vi "Main.vi"() -> ()   [LabVIEW 2019]
uses:
  Typedefs/#enum_MasterState.ctl
  Typedefs/#cluster_GUIRefs.ctl
  SubVIs/LowLevelError.vi
panel:
  in  "Results Viewer":bool
  in  "POX Data History":string[](array[string])
  in  "Save?":bool caption="Save Results?"
  in  "Measure":bool
  in  "Measurement Directory":path
  in  "Stop":bool
  out "O2 Saturation":dbl(graph)
  out "Heart beat":dbl(graph)
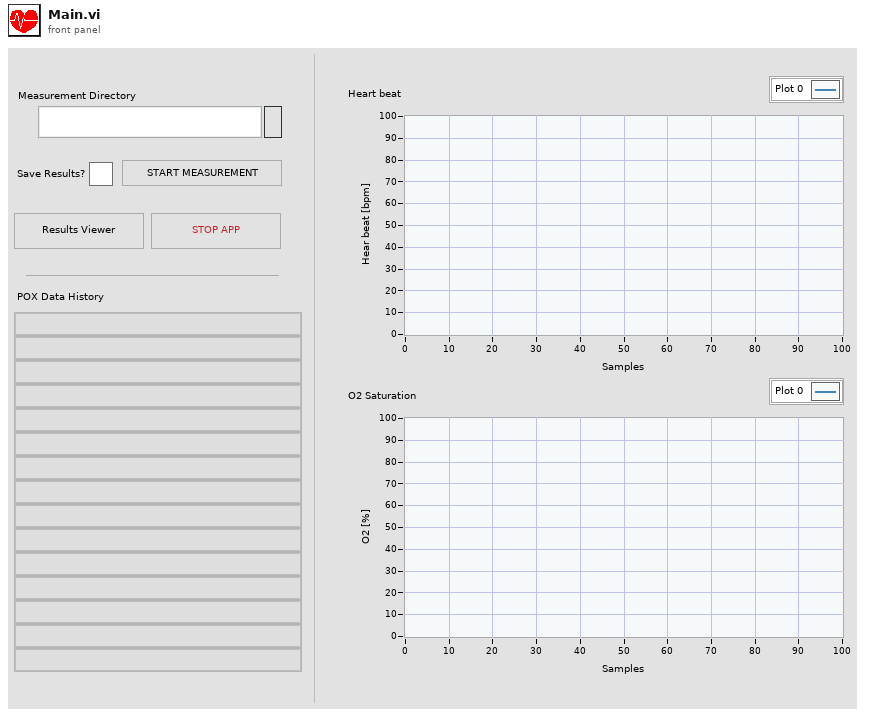
[diagram p1: front panel]
types:
  T1 = typedef "#enum_MasterState.ctl" = enum16{"Idle", "Init", "Close", "Error"}
  T2 = typedef "#cluster_ApplicationData.ctl" = cluster{"Acq Queue":refnum<queue>, "Saving Queue":refnum<queue>}
  T3 = typedef "#cluster_GUIRefs.ctl" = cluster{"Measure":refnum<vi>, "Save?":refnum<vi>, "Stop":refnum<vi>, "Measurement Dir":refnum<vi>, "Heart beat":refnum<vi>, "O2":refnum<vi>, "POX Data History":refnum<vi>}
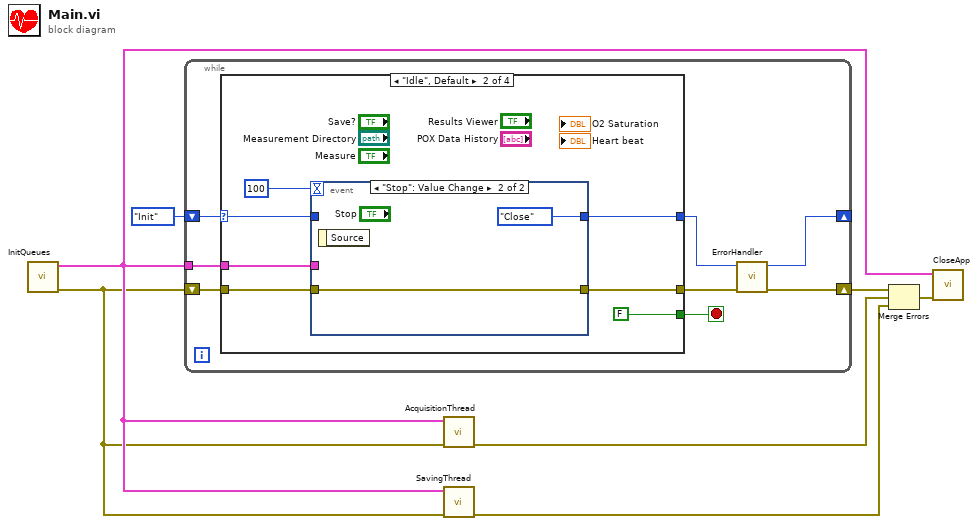
[diagram p0: block diagram]
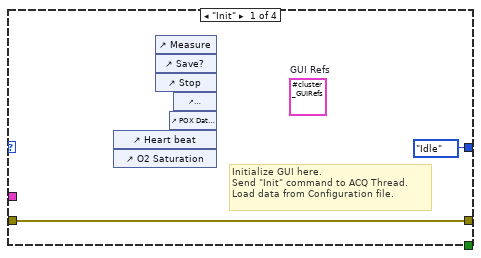
[diagram p2: hidden frame]
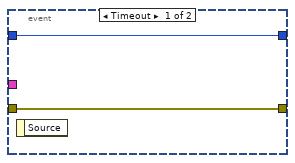
[diagram p3: hidden frame]
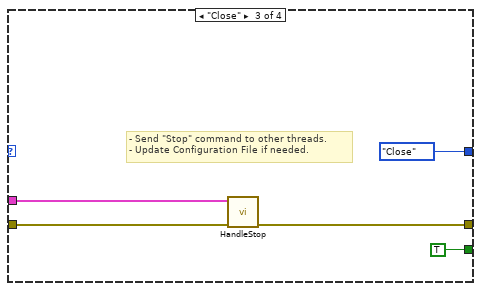
[diagram p4: hidden frame]
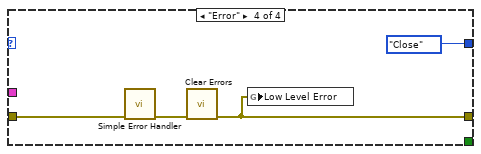
[diagram p5: hidden frame]
diagram:
  n1 = call "InitQueues.vi"() -> ("error out"=w2:errorcluster, "Application Data"=w3:T2)  [unwired: 10 in]
  n2 = while {
    tunnel: w3 -> [w14]
    shift-right: [w10] -> w7
    shift-left: w2 -> [w15]
    shift-right: [w8] -> _
    shift-left: #enum_MasterState."Init" ("Master State") -> [w12]
    stop <- w13 stop-if-true
    n3 = case shown="\"Idle\", Default" w12 {
      selector: w12 -> [_ w21 _ _]
      tunnel: w15 -> [w17 w24 w31 w36]
      tunnel: w14 -> [_ w23 w30 _]
      tunnel: [w17 w22 w29 w34] -> w11
      tunnel: [_ FALSE TRUE _] -> w13
      tunnel: [#enum_MasterState."Idle" ("Master State") w20 #enum_MasterState."Close" ("Master State") #enum_MasterState."Close" ("Master State")] -> w9
      frame "Init" {
        (unwired) T3 {"Measure"=refnum, "Save?"=refnum, "Stop"=refnum, "Measurement Dir"=refnum, "Heart beat"=refnum, "O2"=refnum, "POX Data History"=refnum}  # GUI Refs
        # "Initialize GUI here.\nSend \"Init\" command to ACQ Thread.\nLoad data from Configuration file."
        n4 = control-ref of="Heart beat"() -> ()  [unwired: 1 out]
        n5 = control-ref of="O2 Saturation"() -> ()  [unwired: 1 out]
        n6 = control-ref of="Measure"() -> ()  [unwired: 1 out]
        n7 = control-ref of="Save?"() -> ()  [unwired: 1 out]
        n8 = control-ref of="Stop"() -> ()  [unwired: 1 out]
        n9 = control-ref of="POX Data History"() -> ()  [unwired: 1 out]
        n10 = control-ref of="Measurement Directory"() -> ()  [unwired: 1 out]
      }
      frame "Idle", Default {
        n11 = event shown="[1] \"Stop\": Value Change" {
          selector: _ -> [_ _]
          dyn-events: _ -> [_ _]
          timeout: 100 -> [_ _]
          tunnel: w24 -> [w26 w28]
          tunnel: w23 -> [_ _]
          tunnel: [w26 w28] -> w22
          tunnel: w21 -> [w25 _]
          tunnel: [w25 #enum_MasterState."Close" ("Master State")] -> w20
          event Timeout {
            n12 = event-data() -> ()  [unwired: 1 in, 1 out]
          }
          event "Stop": Value Change {
            n13 = event-data() -> ()  [unwired: 1 in, 1 out]
          }
        }
      }
      frame "Close" {
        # "- Send \"Stop\" command to other threads. \n- Update Configuration File if needed."
        n14 = call "HandleStop.vi"("error in (no error)"=w31, "Application Data"=w30) -> ("error out"=w29:errorcluster)  [unwired: 9 in]
      }
      frame "Error" {
        n15 = call <vilib>:"Simple Error Handler.vi"("error in (no error)"=w36) -> ("error out"=w35:errorcluster)  [unwired: 4 in, 4 out]
        n16 = call <vilib>:"Clear Errors.vi"("error in (no error)"=w35) -> ("error out"=w34:errorcluster)  [unwired: 5 in, 1 out]
        n17 = global write "LowLevelError.vi" "Low Level Error"(w34) -> ()
      }
    }
    n18 = call "ErrorHandler.vi"("error in (no error)"=w11, "Master State in"=w9) -> ("error out"=w10:errorcluster, "Master State out"=w8:T1)  [unwired: 8 in]
  }
  n19 = call "AcquisitionThread.vi"("error in (no error)"=w2, "Application Data"=w3) -> ("error out"=w6:errorcluster)  [unwired: 9 in]
  n20 = call "SavingThread.vi"("error in (no error)"=w2, "Application Data"=w3) -> ("error out"=w1:errorcluster)  [unwired: 9 in]
  n21 = Merge Errors(w7, w6, w1) -> (w5:errorcluster)
  n22 = call "CloseApp.vi"("error in (no error)"=w5, "Application Data"=w3) -> ()  [unwired: 9 in, 1 out]
